vi "Packet TX Only.vi"() -> ()   [LabVIEW 2017, in "My Network Host v1.lvlib"]
uses:
  My Network Host v1.lvlib
  <vilib>/userdefined/Silver/nirio_resource_slv.ctl
  <vilib>/Utility/error.llb/Error Cluster From Error Code.vi
  <vilib>/rvi/errors/niLvFpgaAdjustHostInterfaceError.vi
  <vilib>/FPGAPlugInAG/Dynamic/niLvFpga_Close_Dynamic.vi
  <vilib>/rvi/interface/nirviReadWriteControl/nirviReadWriteControl.xnode
  <vilib>/rvi/interface/nirviCloseFPGA/nirviCloseFPGA.xnode
  NiFpgaLv.dll
  <vilib>/rvi/interface/Simulation/niFpgaSimulationCallBeginRW.vi
panel:
  in  "Remote Detection Delay":dbl=5.0 format="%#_3ps"
  out "MAC local address":u8[](array[numeric])=[0, 1, 2, 3, 4, 5] format="%.0x"
  out "error out":errorcluster
  out "MAC destination address":u8[](array[numeric])=[255, 255, 255, 255, 255, 255] format="%.0x"
  in  "send packet":bool
  in  "udp payload length":u16=512
  in  "Local IP Address":string="169.254.122.140"
  in  "Remote IP Address":string="169.254.117.125"
  in  "UDP destination port":u16=1234
  in  "Stop Button":bool
  out "CLIP state":T1
  in  "resource name":T2="RIO0"
  # "FPGA produces data that looks like it is coming from"
  # "Where to send data to"
  # "Instructions\nNote: Compile the \"FPGA Top - Packet TX Only\" FPGA Target before running this VI. Error 7 \"File not found\" most likely means the bitfile has not been compiled yet.\n\n1. Configure \"Local IP Address\" for the IP you wish the FPGA to have\n2. Configure \"Remote IP Address\" for the IP of the receiving PC or device\n3. Start a program monitoring \"UDP destination port\" on the receiver\n4. Run the VI.  Click \"send packet\" to transmit \"udp payload length\" of zeros (the simulated payload in the example)."
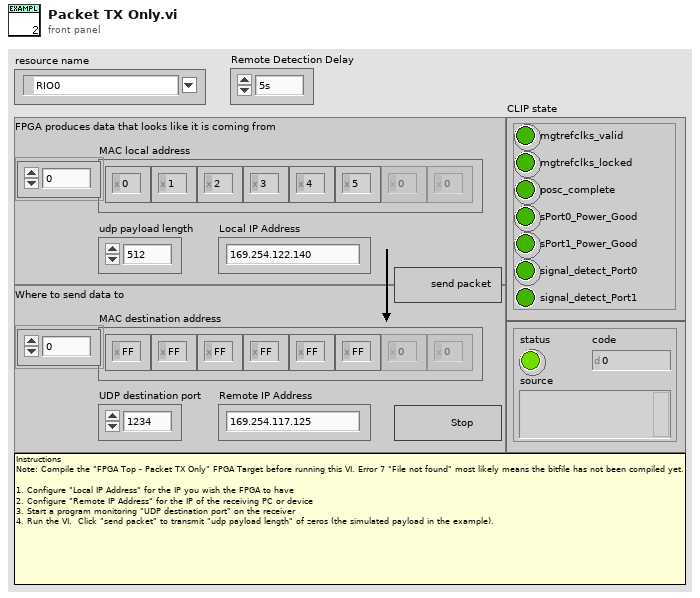
[diagram p1: front panel]
types:
  T1 = cluster{"mgtrefclks_valid":bool, "mgtrefclks_locked":bool, "posc_complete":bool, "sPort0_Power_Good":bool, "sPort1_Power_Good":bool, "signal_detect_Port0":bool, "signal_detect_Port1":bool}
  T2 = typedef "nirio_resource_slv.ctl" = tag
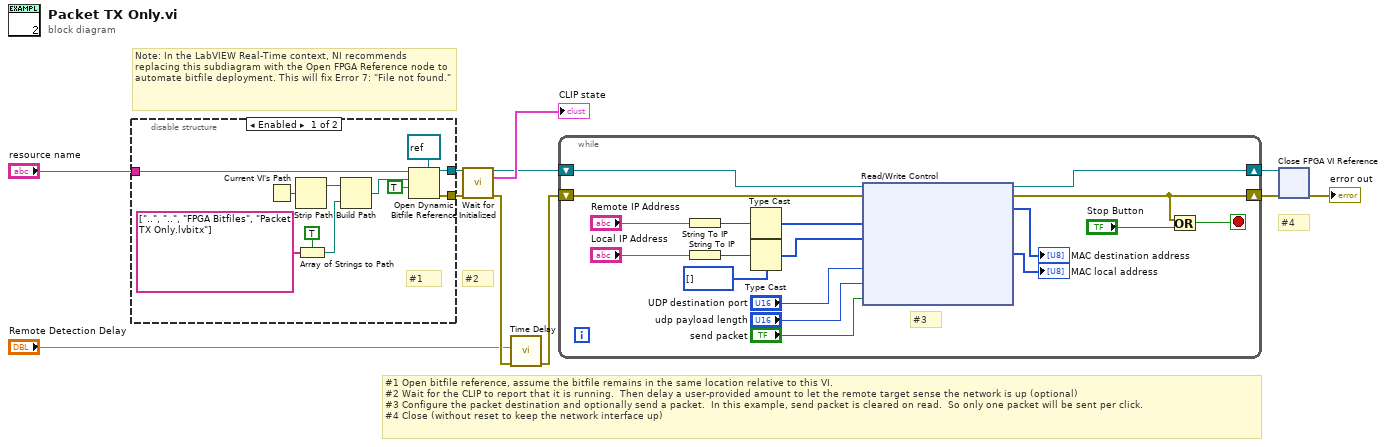
[diagram p0: block diagram]
diagram:
  # "Note: In the LabVIEW Real-Time context, NI recommends replacing this subdiagram with the Open FPGA Reference node to automate bitfile deployment. This will fix Error 7: \"File not found.\""
  # "#4"
  # "#2"
  # "#1 Open bitfile reference, assume the bitfile remains in the same location relative to this VI.\n#2 Wait for the CLIP to report that it is running.  Then delay a user-provided amount to let the remote target sense the network is up (optional)\n#3 Configure the packet destination and optionally send a packet.  In this example, send packet is cleared on read.  So only one packet will be sent per click.\n#4 Close (without reset to keep the network interface up)"
  n1 = disable-structure shown="Enabled" {
    disable-tunnel: "resource name" -> [w22 _]
    disable-tunnel: [w21 _] -> w10
    disable-tunnel: [w20 _] -> w4
    frame Enabled {
      # "#1"
      n2 = Current VI's Path() -> (path=w17:path)
      n3 = Strip Path(path=w17) -> (stripped path=w12:path)  [unwired: 1 out]
      n4 = Array of Strings to Path(0:string[] ["..", "..", "FPGA Bitfiles", "Packet TX Only.lvbitx"] ("array of strings"), 1:TRUE ("relative")) -> (2:w13:path)
      n5 = Build Path(base path=w12, name or relative path=w13) -> (appended path=w16:path)
      n6 = Open Dynamic Bitfile Reference(0:w22, 1:w16, 2:TRUE ("Run When Loaded"), 4:refnum<k20> refnum ("FPGA VI Reference Out")) -> (5:w20:refnum<k20>, 8:w21:errorcluster)  [unwired: 1 in]
    }
    frame Disabled {
      # "Insert code here for LabVIEW Real-Time"
    }
  }
  n7 = call "Wait for Initialized.vi"("Refnum in"=w4, "error in (no error)"=w10) -> ("Refnum out"=w8:refnum<k20>, "CLIP state"=→"CLIP state":T1, "error out"=w3:errorcluster)  [unwired: 11 in]
  n8 = call "Time Delay"("error in (no error)"=w3, "Delay Time (s)"="Remote Detection Delay") -> ("error out"=w2:errorcluster)  [unwired: 9 in]
  n9 = while {
    shift-right: [w39] -> w7
    shift-left: w8 -> [w40]
    shift-right: [w35] -> w6
    shift-left: w2 -> [w38]
    stop <- w36 stop-if-true
    w29 = u8[] [] ("*(type *) &x")
    # "#3"
    n10 = String To IP(1:"Remote IP Address") -> (0:w33:u32)
    n11 = String To IP(1:"Local IP Address") -> (0:w32:u32)
    n12 = Type Cast(type=w29, x=w33) -> (*(type *) &x=w30:u8[])
    n13 = Type Cast(type=w29, x=w32) -> (*(type *) &x=w28:u8[])
    n14 = xnode "Read/Write Control"("FPGA VI Reference In"=w40, "error in"=w38, "IPv4 destination address"=w30, "IPv4 source address"=w28, "UDP destination port"="UDP destination port", "udp payload length"="udp payload length", "send packet"="send packet") -> ("FPGA VI Reference Out"=w39:refnum<k20>, "error out"=w35:errorcluster, "MAC destination address"=→"MAC destination address":u8[], "MAC source address"=→"MAC local address":u8[])
    n15 = Or(x=w35, y="Stop Button") -> (x .or. y?=w36:bool)
  }
  n16 = xnode "Close FPGA VI Reference"("FPGA VI Reference In"=w7, "error in"=w6) -> ("error out"=→"error out":errorcluster)
